vi "KE2602 Config voltage and measure current.vi"(3 "Error Query (False)":bool, 4 "Limit":dbl=1.0, 5 "Measure Function (Current)":T1(ring), 6 "Level":dbl=1.0, 7 "Source Function (Current)":enum32{"Current", "Voltage"}(ring)=enum."Voltage", 8 "error in (no error)":errorcluster, 9 "Channel (Channel A)":T2, 10 "Node (0-64)":i8 min=0 max=64 step=1, 11 "VISA resource name":refnum<visa-resource-name>) -> (0 "error out":errorcluster, 1 "Output":string)   [LabVIEW 2013]
doc: "This example shows how to configure the source and take a measurement."
uses:
  <instrlib>/Keithley 2600 Series/Public/Channel.ctl
  <instrlib>/Keithley 2600 Series/Keithley 2600 Series.lvlib
panel:
  in  "stop":bool
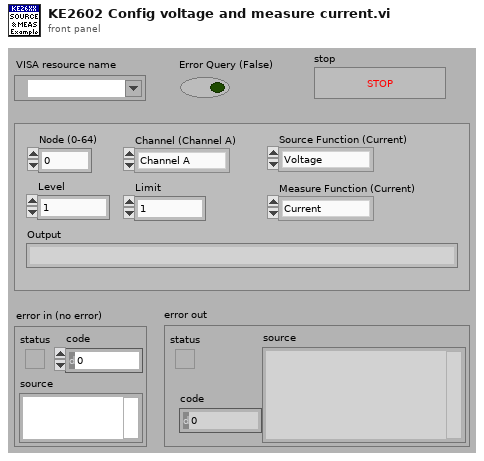
[diagram p1: front panel]
types:
  T1 = enum32{"Current", "Voltage", "IV", "Resistance", "Power"}
  T2 = typedef "Keithley 2600 Series.lvlib/Channel.ctl" = enum32{"Channel A", "Channel B"}
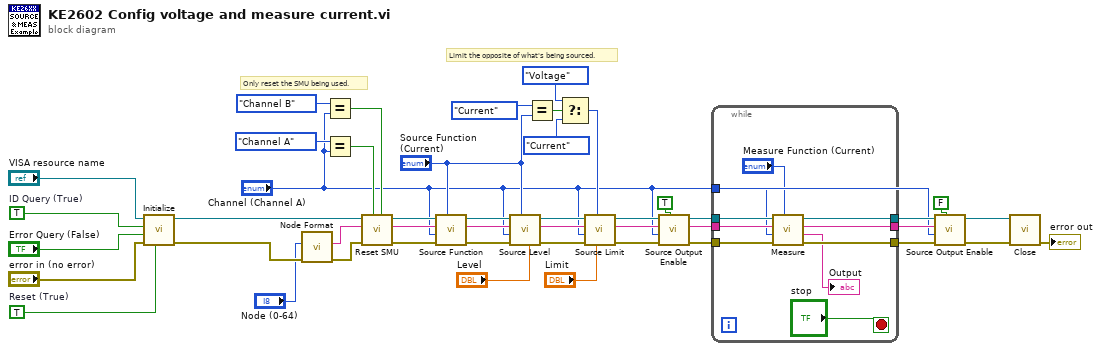
[diagram p0: block diagram]
diagram:
  w14 = TRUE  # Reset (True)
  w44 = TRUE  # ID Query (True)
  # "Limit the opposite of what's being sourced."
  # "Only reset the SMU being used."
  n1 = call <instrlib>:"Initialize.vi"("Reset (True)"=w14, "error in (no error)"="error in (no error)", "Error Query (False)"="Error Query (False)", "ID Query (True)"=w44, "VISA resource name"="VISA resource name") -> ("error out"=w4:errorcluster, "VISA resource name out"=w42:refnum<visa-resource-name>)  [unwired: 1 in, 4 out]
  n2 = call <instrlib>:"Node Format.vi"("error in"=w4, "Node (0-64)"="Node (0-64)") -> ("error out"=w3:errorcluster, "Formatted Node"=w5:string)  [unwired: 8 out]
  n3 = Equal?(x=enum32{"Channel A", "Channel B"}."Channel B", y="Channel (Channel A)") -> (x = y?=w38:bool)
  n4 = Equal?(x=enum32{"Channel A", "Channel B"}."Channel A", y="Channel (Channel A)") -> (x = y?=w39:bool)
  n5 = call <instrlib>:"Reset SMU.vi"("SMU B (No)"=w38, "SMU A (No)"=w39, "error in (no error)"=w3, "Node In"=w5, "VISA resource name"=w42) -> ("error out"=w37:errorcluster, "Node Out"=w35:string, "VISA resource name out"=w36:refnum<visa-resource-name>)  [unwired: 4 out]
  n6 = call <instrlib>:"Source Function.vi"("Function (Current)"="Source Function (Current)", "error in (no error)"=w37, "Channel (Channel A)"="Channel (Channel A)", "Node In"=w35, "VISA resource name"=w36) -> ("error out"=w32:errorcluster, "Node Out"=w34:string, "VISA resource name out"=w33:refnum<visa-resource-name>)  [unwired: 4 out]
  n7 = call <instrlib>:"Source Level.vi"("Level (0.000)"="Level", "Function (Current)"="Source Function (Current)", "error in (no error)"=w32, "Channel (Channel A)"="Channel (Channel A)", "Node In"=w34, "VISA resource name"=w33) -> ("error out"=w31:errorcluster, "Node Out"=w18:string, "VISA resource name out"=w30:refnum<visa-resource-name>)  [unwired: 3 out]
  n8 = Equal?(x=enum32{"Current", "Voltage"}."Current", y="Source Function (Current)") -> (x = y?=w11:bool)
  n9 = Select(t=enum32{"Current", "Voltage"}."Voltage" ("x"), s=w11, f=enum32{"Current", "Voltage"}."Current") -> (s? t:f=w9:enum32{"Current", "Voltage"})
  n10 = call <instrlib>:"Source Limit.vi"("Limit (0.000)"="Limit", "Function (Current)"=w9, "error in (no error)"=w31, "Channel (Channel A)"="Channel (Channel A)", "Node In"=w18, "VISA resource name"=w30) -> ("error out"=w28:errorcluster, "Node Out"=w17:string, "VISA resource name out"=w29:refnum<visa-resource-name>)  [unwired: 3 out]
  n11 = call <instrlib>:"Source Output Enable.vi"("Output (Off)"=TRUE, "error in (no error)"=w28, "Channel (Channel A)"="Channel (Channel A)", "Node In"=w17, "VISA resource name"=w29) -> ("error out"=w27:errorcluster, "Node Out"=w16:string, "VISA resource name out"=w26:refnum<visa-resource-name>)  [unwired: 4 out]
  n12 = while {
    tunnel: w27 -> [w56]
    tunnel: w26 -> [w55]
    tunnel: [w54] -> w25
    tunnel: [w53] -> w24
    tunnel: w16 -> [w52]
    tunnel: [w51] -> w15
    tunnel: "Channel (Channel A)" -> [w49]
    stop <- "stop" stop-if-true
    n13 = call <instrlib>:"Measure.vi"("Function (Current)"="Measure Function (Current)", "error in (no error)"=w56, "Channel (Channel A)"=w49, "Node In"=w52, "VISA resource name"=w55) -> ("error out"=w53:errorcluster, "Output"=→"Output":string, "Node Out"=w51:string, "VISA resource name out"=w54:refnum<visa-resource-name>)  [unwired: 2 in, 1 out]
  }
  n14 = call <instrlib>:"Source Output Enable.vi"("Output (Off)"=FALSE, "error in (no error)"=w24, "Channel (Channel A)"="Channel (Channel A)", "Node In"=w15, "VISA resource name"=w25) -> ("error out"=w23:errorcluster, "VISA resource name out"=w22:refnum<visa-resource-name>)  [unwired: 5 out]
  n15 = call <instrlib>:"Close.vi"("error in (no error)"=w23, "VISA resource name"=w22) -> ("error out"=→"error out":errorcluster)  [unwired: 9 out]
